vi "stringarray_to_Javascript_variable.vi"(7 "quote":bool, 8 "Array":string[](array[string]), 10 "variable_name":string) -> (0 "variable_string":string)   [LabVIEW 2013]
doc: "Converts an array of stings to a javscript array given by the name.\nQuoting is can be done here if the stings are not quoted already.\nNot safe if the string contains a double quote. \""
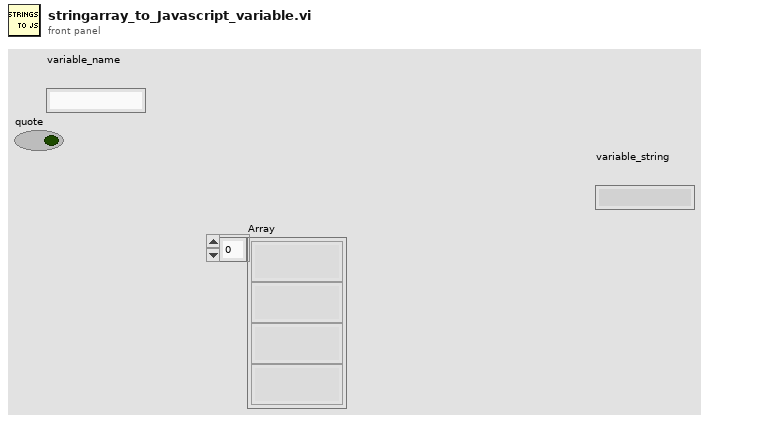
[diagram p1: front panel]
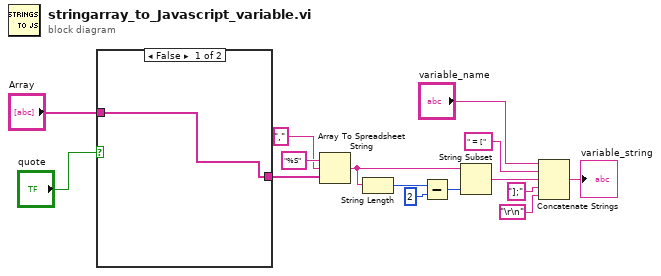
[diagram p0: block diagram]
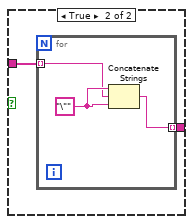
[diagram p2: hidden frame]
diagram:
  n1 = case shown="False" "quote" {
    tunnel: "Array" -> [w16 w18]
    tunnel: [w16 w17] -> w2
    frame False {
    }
    frame True {
      n2 = for {
        tunnel: w18 -> [w20] mode=indexing
        tunnel: [w19] -> w17 mode=indexing
        w21 = "\"" ("string")
        n3 = Concatenate Strings(w21, w20, w21) -> (w19:string)
      }
    }
  }
  n4 = Array To Spreadsheet String(delimiter (Tab)="," ("string"), array=w2, 3:"%S" ("format string")) -> (spreadsheet string=w9:string)
  n5 = String Length(string=w9) -> (length=w10:i32)
  n6 = Subtract(x=w10, y=2) -> (x-y=w11:i32)
  n7 = String Subset(string=w9, length (rest)=w11) -> (substring=w6:string)  [unwired: 1 in]
  n8 = Concatenate Strings("variable_name", " = [", w6, "];", "\r\n") -> (→"variable_string":string)
